vi "配置写入.vi"(8 "error in (no error)":errorcluster caption="错误输入（无错误）", 11 "数据值":T1 {"配置信息"."定点周期"."时间" items=["00:00", "01:00", "02:00", "03:00", "04:00", "05:00", "06:00", "07:00", "08:00", "09:00", "10:00", "11:00", "12:00", "13:00", "14:00", "15:00", "16:00", "17:00", "18:00", "19:00", "20:00", "21:00", "22:00", "23:00"]}) -> (0 "error out":errorcluster caption="错误输出")   [LabVIEW 2016, in "TimingControl.lvlib" / "TimingControl.lvclass"]
uses:
  TimingControl.lvclass
  State Data.ctl
  <vilib>/Utility/xml.llb/Write to XML File(string).vi
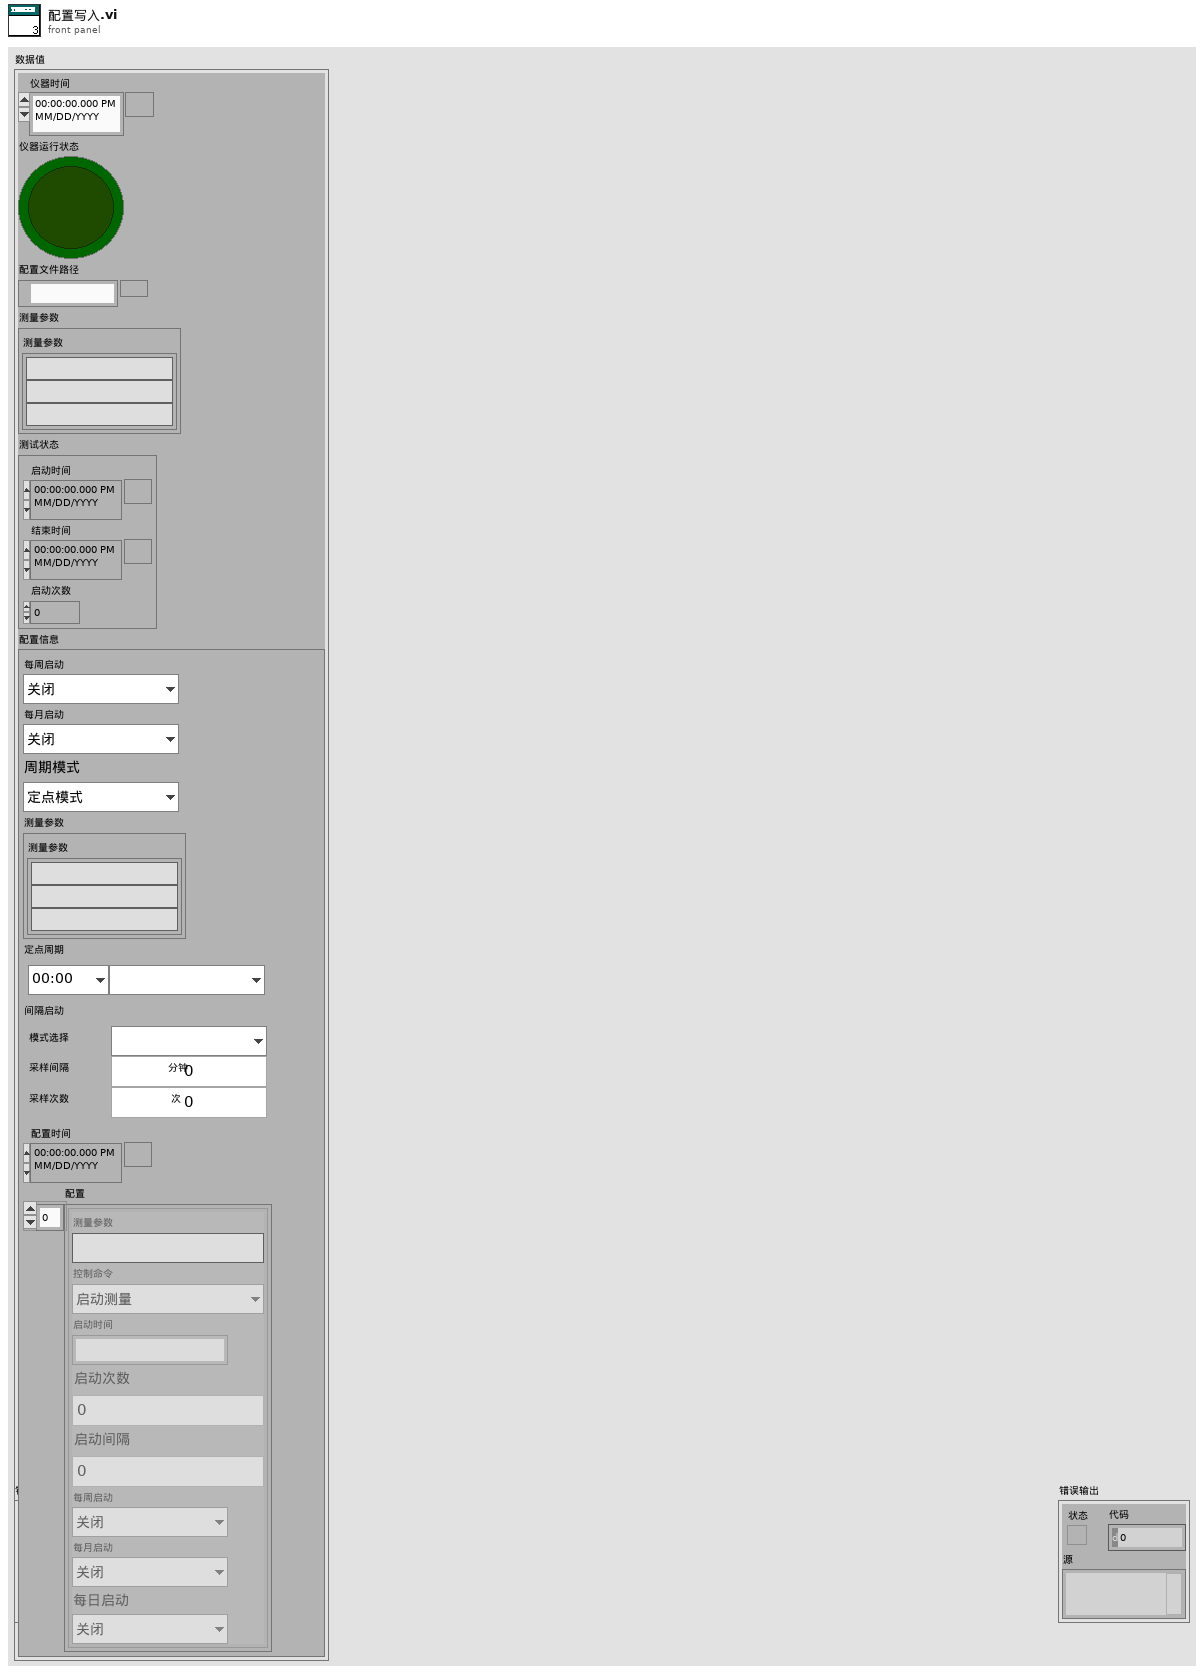
[diagram p1: front panel]
types:
  T1 = typedef "TimingControl.lvlib/TimingControl.lvclass/State Data.ctl" = cluster{"仪器时间":timestamp, "仪器运行状态":bool, "配置文件路径":path, "测量参数":T2, "测试状态":cluster{"启动时间":timestamp, "结束时间":timestamp, "启动次数":i32}, "配置信息":T3}
  T2 = typedef "TimingControl.lvlib/TimingControl.lvclass/测量参数.ctl" = cluster{"测量参数":string[]}
  T3 = typedef "TimingControl.lvlib/TimingControl.lvclass/配置信息.ctl" = cluster{"每周启动":T4, "每月启动":T5, "周期模式":T6, "测量参数":T2, "定点周期":T7, "间隔启动":T9, "配置时间":timestamp, "配置":cluster{"测量参数":string, "控制命令":T10, "启动时间":string, "启动次数":u16, "启动间隔":dbl, "每周启动":T4, "每月启动":T5, "每日启动":enum16{"关闭", "每日"}}[]}
  T4 = typedef "TimingControl.lvlib/TimingControl.lvclass/每周启动.ctl" = enum16{"关闭", "周日", "周一", "周二", "周三", "周四", "周五", "周六"}
  T5 = typedef "TimingControl.lvlib/TimingControl.lvclass/每月启动.ctl" = enum16{"关闭", "1号", "2号", "3号", "4号", "5号", "6号", "7号", "8号", "9号", "10号", "11号", "12号", "13号", "14号", "15号", "16号", "17号", "18号", "19号", "20号", "21号", "22号", "23号", "24号", "25号", "26号", "27号", "28号", "29号", "30号", "31号"}
  T6 = typedef "TimingControl.lvlib/TimingControl.lvclass/周期模式设置.ctl" = enum16{"定点模式", "间隔模式"}
  T7 = typedef "TimingControl.lvlib/TimingControl.lvclass/定点周期设置.ctl" = cluster{"时间":u16, "启动命令":T8}
  T8 = typedef "TimingControl.lvlib/TimingControl.lvclass/启动命令选择.ctl" = enum16{"", "水样测试", "标样核查", "零点核查", "跨度核查", "空白测试", "平行样测试", "加标回收", "空白校准", "标样校准", "初始化(清洗)"}
  T9 = typedef "TimingControl.lvlib/TimingControl.lvclass/间隔启动设置.ctl" = cluster{"启动命令":T8, "启动间隔":dbl, "启动次数":i32}
  T10 = typedef "TimingControl.lvlib/TimingControl.lvclass/国标控制命令.ctl" = enum16{"启动测量", "标样核查", "零点核查", "跨度核查", "空白测试", "平行样测试", "加标回收", "空白校准", "标样校准", "初始化（清洗）", "停止测试", "仪器重启", "校时", "模式设置", "测量间隔设置"}
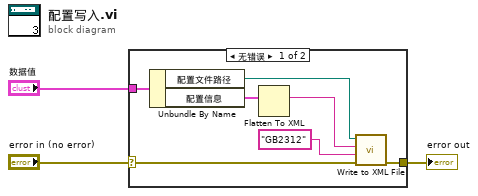
[diagram p0: block diagram]
diagram:
  n1 = case shown="无错误" "error in (no error)" {
    selector: "error in (no error)" -> [w8 w11]
    tunnel: [w7 w11] -> w2
    tunnel: "数据值" -> [w6 _]
    frame No Error {
      n2 = Unbundle By Name(w6) -> ("配置文件路径"=w4:path, "配置信息"=w5:T3)
      n3 = Flatten To XML(anything=w5) -> (xml string=w10:string)
      n4 = call-poly <vilib>:"Write to XML File.vi"("error in (no error)"=w8, "XML Encoding"="GB2312", "XML Input"=w10, "XML File Path"=w4) -> ("error out"=w7:errorcluster)  [unwired: 5 in, 2 out]
    }
    frame Error {
    }
  }
  "error out" <- w2
